vi "9607 Invalid Cast--error.vi"(8 "error in":errorcluster, 10 "Value":i32, 11 "Type":string) -> (0 "error out":errorcluster)   [LabVIEW 2024, in "Electronic Datasheet.lvlib"]
uses:
  Electronic Datasheet.lvlib
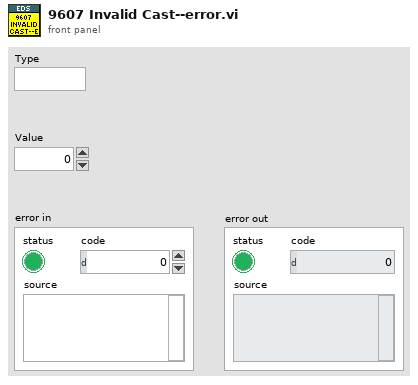
[diagram p1: front panel]
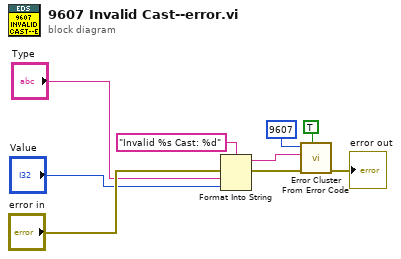
[diagram p0: block diagram]
diagram:
  n1 = Format Into String(format string="Invalid %s Cast: %d" ("error message (\"\")"), error in="error in", "Type", "Value") -> (resulting string=w8:string, error out=w3:errorcluster)  [unwired: 1 in]
  n2 = call <vilib>:"Error Cluster From Error Code.vi"("show call chain? (False)"=TRUE, "error in (no error)"=w3, "error message (\"\")"=w8, "error code (0)"=9607) -> ("error out"=→"error out":errorcluster)  [unwired: 5 in]
